vi "Search for time to keep.vi"(9 "newest time to keep":u64, 10 "oldest time to keep":u64, 11 "timestamps (incrementing)":u64[](array[numeric])) -> (1 "length":i32, 2 "index":i32, 3 "timestamps (dup)":u64[](array[numeric]))   [LabVIEW 2021, in "Ring Buffer Strict Accessor.lvlib"]
uses:
  Ring Buffer Strict Accessor.lvlib
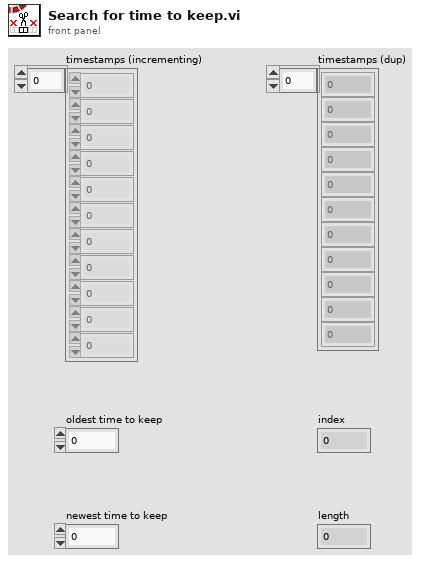
[diagram p1: front panel]
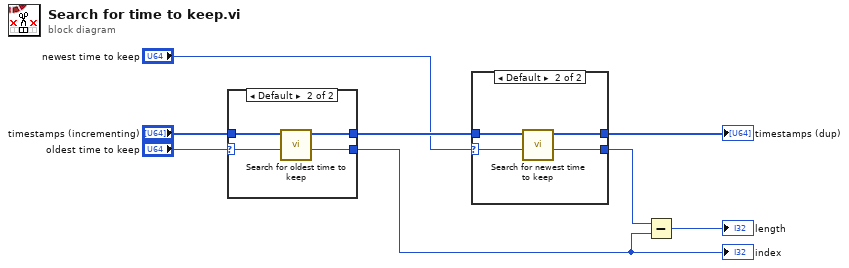
[diagram p0: block diagram]
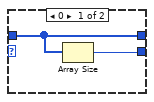
[diagram p3: hidden frame]
diagram:
  n1 = case shown="Default" "oldest time to keep" {
    selector: "oldest time to keep" -> [_ w11]
    tunnel: "timestamps (incrementing)" -> [w9 w13]
    tunnel: [w9 w12] -> w7
    tunnel: [_ w10] -> w3
    frame 0 {
    }
    frame Default {
      n2 = call "Search for oldest time to keep.vi"("oldest time to keep"=w11, "timestamps (incrementing)"=w13) -> ("split index"=w10:i32, "timestamps (dup)"=w12:u64[])  [unwired: 8 in]
    }
  }
  "index" <- w3
  n3 = case shown="Default" "newest time to keep" {
    selector: "newest time to keep" -> [_ w18]
    tunnel: w7 -> [w15 w19]
    tunnel: [w15 w17] -> w4
    tunnel: [w14 w16] -> w1
    frame 0 {
      n4 = Array Size(array=w15) -> (size(s)=w14:i32)
    }
    frame Default {
      n5 = call "Search for newest time to keep.vi"("newest time to keep"=w18, "timestamps (incrementing)"=w19) -> ("split index"=w16:i32, "timestamps (dup)"=w17:u64[])  [unwired: 8 in]
    }
  }
  "timestamps (dup)" <- w4
  n6 = Subtract(x=w1, y=w3) -> (x-y=→"length":i32)
